vi "temp_monitor.vi"() -> ()   [LabVIEW 2017]
uses:
  istr.lib/Keithley 2100 Series/Public/Configure/Configure Temperature.vi
  istr.lib/Keithley 2100 Series/Keithley 2100 Series.lvlib
panel:
  out "Measurement":dbl format="%#_6e"
  out "XYグラフ":cluster{timestamp[], dbl[]}(graph)={[timestamp(3738019839.37396 s since 1904-01-01), timestamp(3738019841.369872 s since 1904-01-01), timestamp(3738019842.159289 s since 1904-01-01), timestamp(3738019843.186232 s since 1904-01-01), timestamp(3738019844.211117 s since 1904-01-01), timestamp(3738019845.4481034 s since 1904-01-01)], [24.6260528, 24.6260528, 24.6276672, 24.6292784, 24.6292784, 24.6292784]}
  out "error out":errorcluster
  in  "停止":bool
  in  "COMMENT":string="temerature_configuration_1"
  in  "base path":path=path "C:/LabVIEW/DATA/J-PARC_202206"
  in  "VISA resource name":refnum<visa-resource-name>="USB0::0x05E6::0x2100::8012800::INSTR"
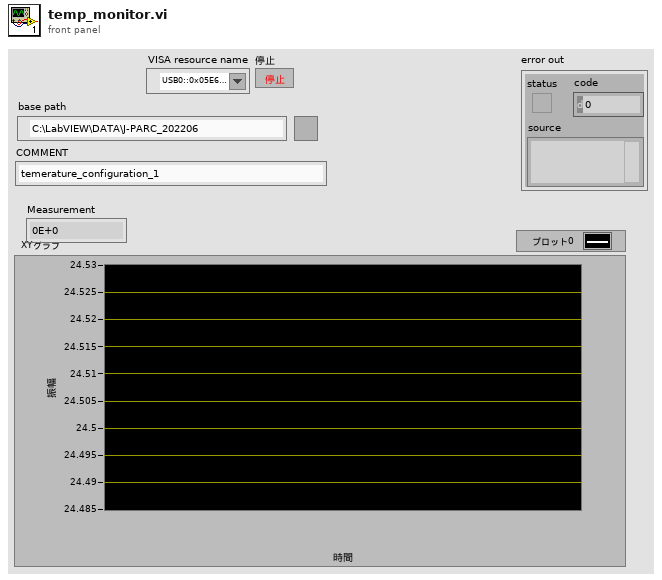
[diagram p1: front panel]
types:
  T1 = enum16{"open", "replace", "create", "open or create", "replace or create", "replace or create with confirmation"}
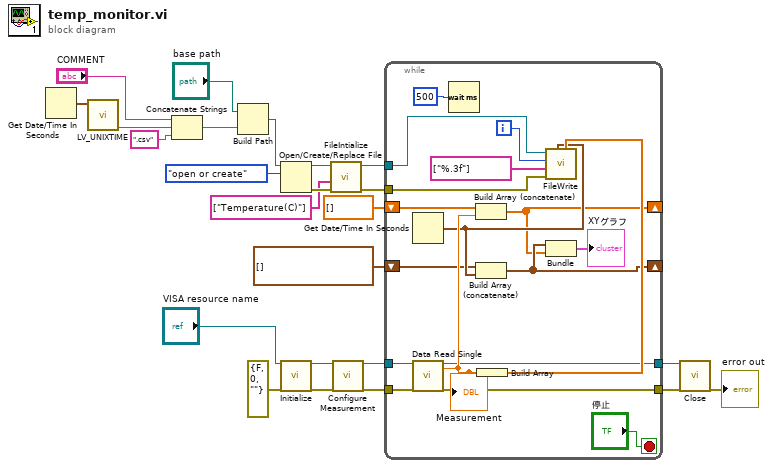
[diagram p0: block diagram]
diagram:
  n1 = Get Date/Time In Seconds() -> (seconds since 1Jan1904=w18:timestamp)
  n2 = call "LV_UNIXTIME.vi"("current time"=w18) -> ("date/time string"=w15:string)  [unwired: 9 in, 1 out]
  n3 = Concatenate Strings("COMMENT", w15, ".csv" ("string")) -> (w13:string)
  n4 = Build Path(base path="base path", name or relative path=w13) -> (appended path=w17:path)
  n5 = Open/Create/Replace File(file path (use dialog)=w17, operation (0:open)=T1."open or create") -> (refnum out=w10:refnum<file>, error out=w11:errorcluster)  [unwired: 4 in, 1 out]
  n6 = call "Initialize.vi"("VISA resource name"="VISA resource name", "error in (no error)"=errorcluster {"status"=FALSE, "code"=0, "source"=""}) -> ("VISA resource name out"=w23:refnum<visa-resource-name>, "error out"=w21:errorcluster)  [unwired: 16 in]
  n7 = call "FileIntialize.vi"("Error In"=w11, "Labels"=string[] ["Temperature(C)"], "refnum in"=w10) -> ("Error Out"=w6:errorcluster, "File Refnum"=w7:refnum<file>)  [unwired: 7 in]
  n8 = call-poly "Configure Measurement.vi"("VISA resource name"=w23, "error in (no error)"=w21) -> ("VISA resource name out"=w8:refnum<visa-resource-name>, "error out"=w20:errorcluster)  [unwired: 16 in]
  n9 = while {
    tunnel: w20 -> [w42]
    tunnel: w8 -> [w40]
    tunnel: w7 -> [w39]
    tunnel: w6 -> [w38]
    shift-right: [w26] -> _
    shift-left: dbl[] [] -> [w31]
    shift-right: [w27] -> _
    shift-left: timestamp[] [] -> [w30]
    tunnel: [w29] -> w3
    tunnel: [w28] -> w2
    i -> [w36]
    stop <- "停止" stop-if-true
    n10 = Get Date/Time In Seconds() -> (seconds since 1Jan1904=w33:timestamp)
    n11 = call "Data Read Single.vi"("VISA resource name"=w40, "error in (no error)"=w42) -> ("VISA resource name out"=w28:refnum<visa-resource-name>, "Measurement"=w34:dbl, "error out"=w29:errorcluster)  [unwired: 15 in]
    "Measurement" <- w34
    n12 = Wait (ms)(milliseconds to wait=u32 500 ("ミリ秒待機時間")) -> ()  [unwired: 1 out]
    n13 = Build Array (concatenate)(w31, w34) -> (w26:dbl[])
    n14 = Build Array (concatenate)(w30, w33) -> (w27:timestamp[])
    n15 = Build Array(w34) -> (w37:dbl[])
    n16 = call "FileWrite.vi"("DataArray"=w37, "Time Stamp"=w33, "Error In"=w38, "FileFormat"=string[] ["%.3f"], "Index"=w36, "refnum in"=w39) -> ()  [unwired: 4 in, 2 out]
    n17 = Bundle(w27, w26) -> (→"XYグラフ":cluster{timestamp[], dbl[]})  [unwired: 1 in]
  }
  n18 = call "Close.vi"("VISA resource name"=w2, "error in (no error)"=w3) -> ("error out"=→"error out":errorcluster)  [unwired: 17 in]
